vi "GetAxisPosition.vi"(0 "Axis":enum16{"Z", "Y", "X"}(ring), 1 "connection refnum in":refnum<k5>, 2 "error in":errorcluster) -> (3 "string result":string, 4 "connection refnum out":refnum<k5>, 5 "numeric result":i32, 6 "error out":errorcluster)   [LabVIEW 2023]
doc: "Get the position of a specificed axis in counts."
uses:
  GlobalVarsNetwork.vi
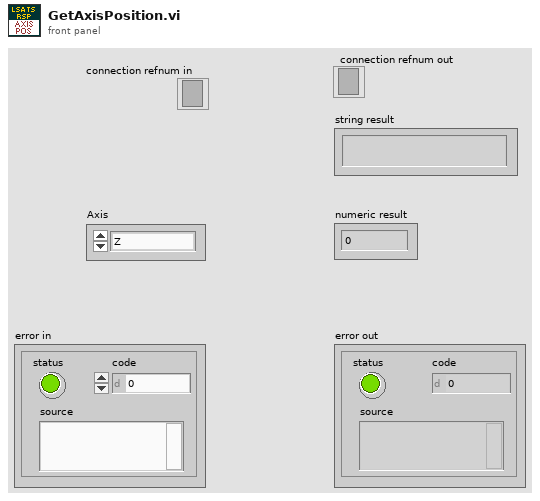
[diagram p1: front panel]
types:
  T1 = cluster{"XY_IP_ADDRESS":string, "Z_IP_ADDRESS":string, "Port":u16, "connection refnum x,y":refnum<k5>, "connection refnum z":refnum<k5>}
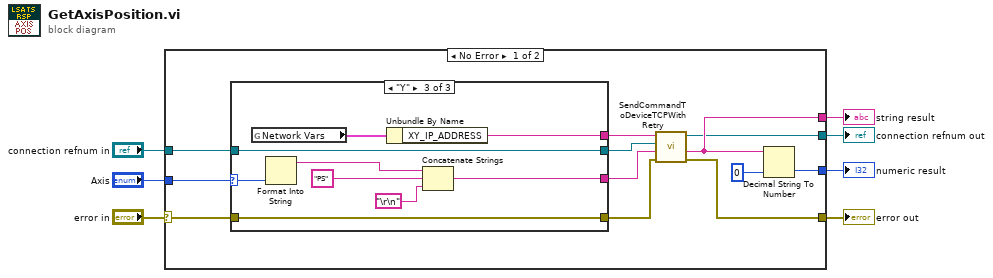
[diagram p0: block diagram]
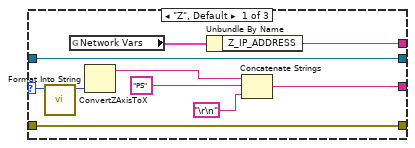
[diagram p2: hidden frame]
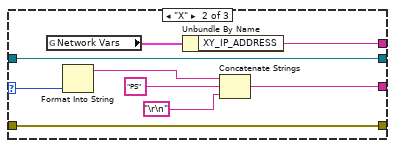
[diagram p3: hidden frame]
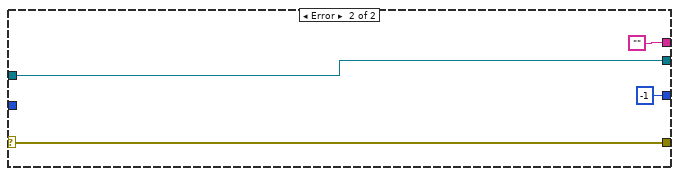
[diagram p4: hidden frame]
diagram:
  n1 = case shown="No Error" "error in" {
    selector: "error in" -> [w12 w51]
    tunnel: "Axis" -> [w19 _]
    tunnel: [w15 w51] -> w6
    tunnel: [w13 ""] -> w5
    tunnel: [w11 -1] -> w3
    tunnel: [w10 w48] -> w2
    tunnel: "connection refnum in" -> [w9 w48]
    frame No Error {
      n2 = case shown="\"Y\"" w19 {
        selector: w19 -> [w22 w33 w44]
        tunnel: [w26 w35 w46] -> w18
        tunnel: [w24 w34 w42] -> w17
        tunnel: w12 -> [w23 w31 w40]
        tunnel: [w23 w31 w40] -> w16
        tunnel: w9 -> [w20 w30 w39]
        tunnel: [w20 w30 w39] -> w8
        frame "Z", Default {
          n3 = call "ConvertZAxisToX.vi"("Axis in"=w22) -> ("Axis out"=w21:enum16{"Z", "Y", "X"})  [unwired: 6 in]
          n4 = global read "GlobalVarsNetwork.vi" "Network Vars"() -> (w29:T1)
          n5 = Format Into String(w21) -> (resulting string=w28:string)  [unwired: 3 in, 1 out]
          n6 = Unbundle By Name(w29) -> ("Z_IP_ADDRESS"=w26:string)
          n7 = Concatenate Strings(w28, "PS", "\r\n") -> (w24:string)
        }
        frame "X" {
          n8 = global read "GlobalVarsNetwork.vi" "Network Vars"() -> (w38:T1)
          n9 = Format Into String(w33) -> (resulting string=w37:string)  [unwired: 3 in, 1 out]
          n10 = Unbundle By Name(w38) -> ("XY_IP_ADDRESS"=w35:string)
          n11 = Concatenate Strings(w37, "PS", "\r\n") -> (w34:string)
        }
        frame "Y" {
          n12 = global read "GlobalVarsNetwork.vi" "Network Vars"() -> (w47:T1)
          n13 = Format Into String(w44) -> (resulting string=w43:string)  [unwired: 3 in, 1 out]
          n14 = Unbundle By Name(w47) -> ("XY_IP_ADDRESS"=w46:string)
          n15 = Concatenate Strings(w43, "PS", "\r\n") -> (w42:string)
        }
      }
      n16 = call "SendCommandToDeviceTCPWithRetry.vi"("error in"=w16, "str command"=w17, "connection refnum in"=w8, "IP address"=w18) -> ("error out"=w15:errorcluster, "str out"=w13:string, "connection refnum out"=w10:refnum<k5>)  [unwired: 4 in, 1 out]
      n17 = Decimal String To Number(string=w13, default (0L)=0 ("default (0 I32)")) -> (number=w11:i32)  [unwired: 1 in, 1 out]
    }
    frame Error {
    }
  }
  "string result" <- w5
  "error out" <- w6
  "numeric result" <- w3
  "connection refnum out" <- w2
